vi "Finish.vi"   [LabVIEW 2014]
doc: "This VI is called just before exiting. It is expected to close I/O refnum, save collected data, etc."
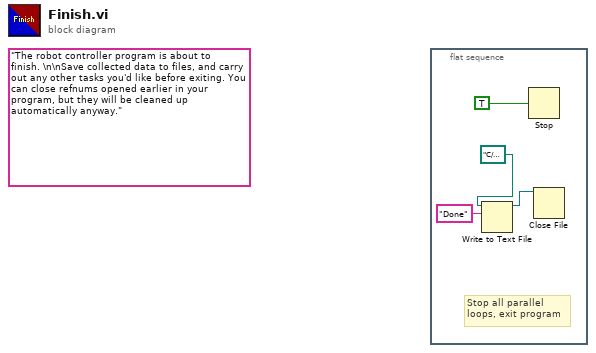
[diagram p0: block diagram]
diagram:
  (unwired) "The robot controller program is about to finish. \n\nSave collected data to files, and carry out any other tasks you'd like before exiting. You can close refnums opened earlier in your program, but they will be cleaned up automatically anyway."
  n1 = flat-sequence {
    frame #0 {
      # "Stop all parallel\nloops, exit program"
      n2 = Write to Text File(file (use dialog)=path "C:/Users/Laura/Documents/Programming/AutonData.txt" ("base path"), text="Done") -> (refnum out=w3:refnum<file>)  [unwired: 2 in, 2 out]
      n3 = Stop(stop? (T)=TRUE ("Quit")) -> ()
      n4 = Close File(refnum=w3) -> ()  [unwired: 1 in, 2 out]
    }
  }
